vi "ControlMotor.vi"(0 "控制电机":T2, 1 "控制电机指令":T3, 2 "位置":T1, 3 "错误输入":errorcluster caption="错误常量", 4 "消息引用":refnum<vi>) -> (8 "错误输出 2":errorcluster caption="输出簇")   [LabVIEW 2018]
panel:
  out "通信成功？":bool
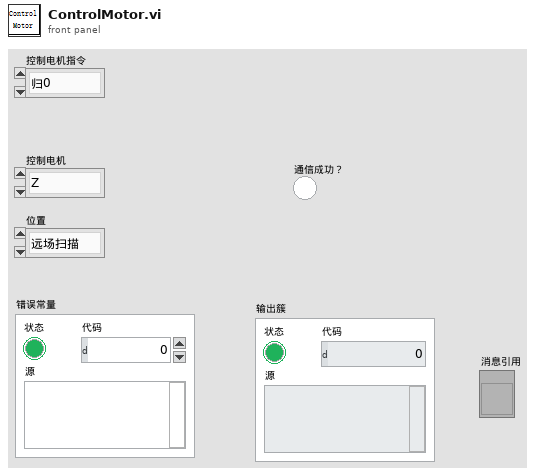
[diagram p1: front panel]
types:
  T1 = typedef "控制电机位置枚举器.ctl" = enum16{"远场扫描", "发散角扫描", "远场相机", "近场相机", "时间波形", "偏振", "能量", "功率", "光谱"}
  T2 = typedef "控制电机枚举器.ctl" = enum16{"Z", "Y", "X", "发散角", "俯仰", "旋转"}
  T3 = typedef "控制电机指令枚举器.ctl" = enum16{"归0", "停止", "运动", "轴设置", "通信连接"}
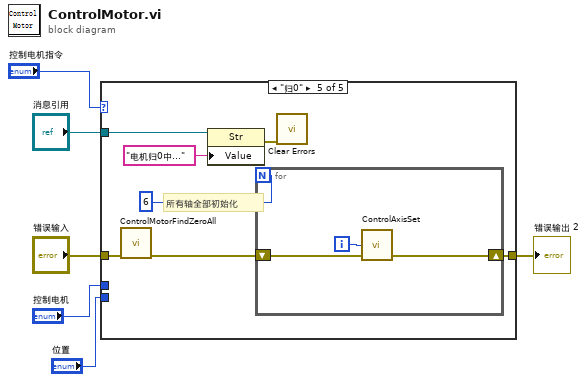
[diagram p0: block diagram]
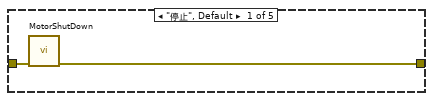
[diagram p2: hidden frame]
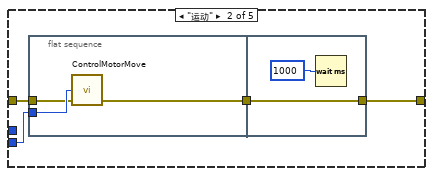
[diagram p3: hidden frame]
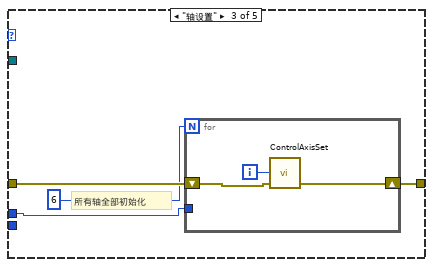
[diagram p4: hidden frame]
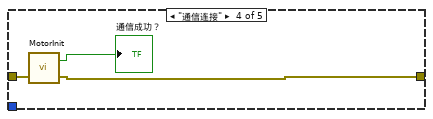
[diagram p5: hidden frame]
diagram:
  n1 = case shown="\"归0\"" "控制电机指令" {
    tunnel: "错误输入" -> [w8 w11 w21 w27 w32]
    tunnel: [w7 w10 w20 w26 w28] -> w4
    tunnel: "控制电机" -> [_ _ w19 _ _]
    tunnel: "位置" -> [_ w12 _ _ _]
    tunnel: "消息引用" -> [_ _ _ _ w34]
    frame "停止", Default {
      n2 = call "MotorShutDown.vi"("error in (no error)"=w8) -> ("error out"=w7:errorcluster)  [unwired: 10 in]
    }
    frame "运动" {
      n3 = flat-sequence {
        tunnel: w12 -> [w15]
        tunnel: w11 -> [w14]
        tunnel: [w13] -> w9
        tunnel: [w17] -> w10
        tunnel: w9 -> [w17]
        frame #0 {
          n4 = call "ControlMotorMove.vi"("错误输入"=w14, "位置"=w15) -> ("错误输出"=w13:errorcluster)  [unwired: 3 in]
        }
        frame #1 {
          n5 = Wait (ms)(milliseconds to wait=u32 1000 ("等待时间（毫秒）")) -> ()  [unwired: 1 out]
        }
      }
    }
    frame "轴设置" {
      # "所有轴全部初始化"
      n6 = for {
        N: 6 -> [_]
        tunnel: w19 -> [_]
        shift-right: [w23] -> w20
        shift-left: w21 -> [w24]
        i -> [w22]
        n7 = call "ControlAxisSet.vi"("错误输入"=w24, "控制电机"=w22) -> ("错误输出"=w23:errorcluster)  [unwired: 3 in]
      }
    }
    frame "通信连接" {
      n8 = call "MotorInit.vi"("错误输入"=w27) -> ("错误输出"=w26:errorcluster, "通信成功？"=→"通信成功？":bool)  [unwired: 1 in]
    }
    frame "归0" {
      # "所有轴全部初始化"
      n9 = call "ControlMotorFindZeroAll.vi"("错误输入"=w32) -> ("error IO"=w29:errorcluster)  [unwired: 10 in]
      n10 = property class="Str"(reference=w34, "Value"="电机归0中..." ("值")) -> (error out=w31:errorcluster)  [unwired: 1 in, 1 out]
      n11 = for {
        N: 6 -> [_]
        shift-right: [w36] -> w28
        shift-left: w29 -> [w37]
        i -> [w35]
        n12 = call "ControlAxisSet.vi"("错误输入"=w37, "控制电机"=w35) -> ("错误输出"=w36:errorcluster)  [unwired: 3 in]
      }
      n13 = call <vilib>:"Clear Errors.vi"("error in (no error)"=w31) -> ()  [unwired: 5 in, 2 out]
    }
  }
  "错误输出 2" <- w4
